vi "Basic Traffic Lights.vi"() -> ()   [LabVIEW 2012]
doc: "VI which is to simply run through the traffic light routine:\nRed -> RedAmber -> Green -> Amber -> Red"
uses:
  Controls/Traffic Light States.ctl
  Controls/Traffic Light Display.ctl
panel:
  in  "Stop Button":bool
  out "Traffic Light Display":T1
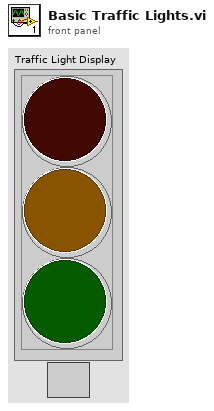
[diagram p1: front panel]
types:
  T1 = typedef "Traffic Light Display.ctl" = cluster{"RED":bool, "AMBER":bool, "GREEN":bool}
  T2 = typedef "Traffic Light States.ctl" = enum16{"Red", "RedAmber", "Green", "Amber"}
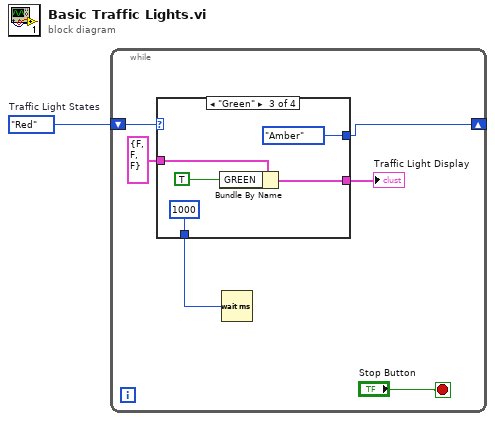
[diagram p0: block diagram]
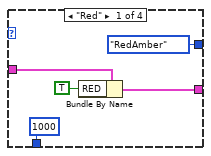
[diagram p2: hidden frame]
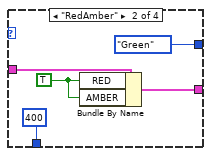
[diagram p3: hidden frame]
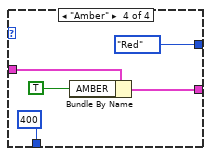
[diagram p4: hidden frame]
diagram:
  w1 = Traffic_Light_States."Red"  # Traffic Light States
  n1 = while {
    shift-right: [w4] -> _
    shift-left: w1 -> [w7]
    stop <- "Stop Button" stop-if-true
    n2 = case shown="\"Green\"" w7 {
      tunnel: T1 {"RED"=FALSE, "AMBER"=FALSE, "GREEN"=FALSE} ("Traffic Light Display") -> [w12 w17 w22 w27]
      tunnel: [w10 w16 w20 w25] -> w5
      tunnel: [Traffic_Light_States."RedAmber" ("Traffic Light States") Traffic_Light_States."Green" ("Traffic Light States") Traffic_Light_States."Amber" ("Traffic Light States") Traffic_Light_States."Red" ("Traffic Light States")] -> w4
      tunnel: [1000 400 1000 400] -> w2
      frame "Red" {
        n3 = Bundle By Name(cluster=w12, "RED"=TRUE) -> (w10:T1)
      }
      frame "RedAmber" {
        w14 = TRUE ("RED")
        n4 = Bundle By Name(cluster=w17, "RED"=w14, "AMBER"=w14) -> (w16:T1)
      }
      frame "Green" {
        n5 = Bundle By Name(cluster=w22, "GREEN"=TRUE ("RED")) -> (w20:T1)
      }
      frame "Amber" {
        n6 = Bundle By Name(cluster=w27, "AMBER"=TRUE ("RED")) -> (w25:T1)
      }
    }
    "Traffic Light Display" <- w5
    n7 = Wait (ms)(milliseconds to wait=w2) -> ()  [unwired: 1 out]
  }
